vi "create TCPReceiver.vi"(8 "error in (no error)":errorcluster, 10 "Packet Type":refnum<class "TCPPacket.lvclass">, 11 "TCPReceiver in":refnum<class "TCPReceiver.lvclass">) -> (0 "error out":errorcluster, 3 "TCPReceiver out":refnum<class "TCPReceiver.lvclass">)   [LabVIEW 2019, in "TCPReceiver.lvclass"]
uses:
  TCPReceiver.lvclass
  TCPPacket/TCPPacket.lvclass
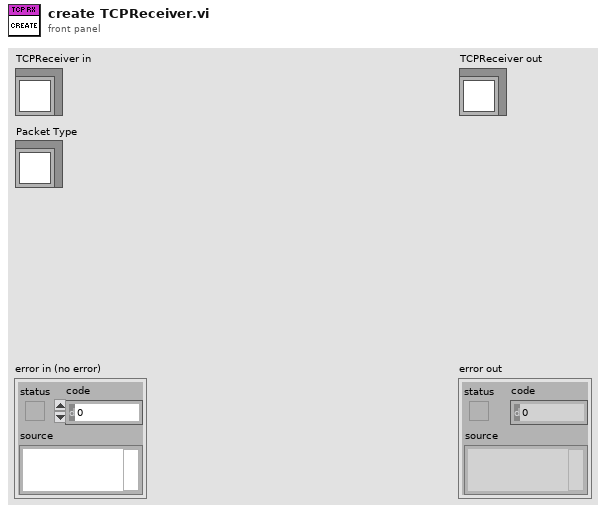
[diagram p1: front panel]
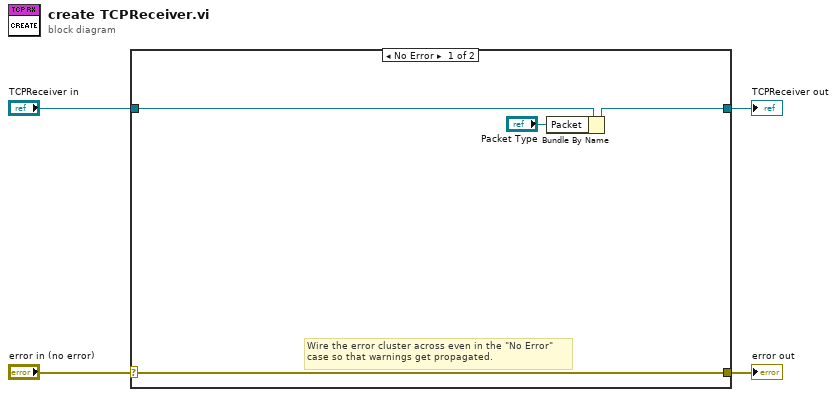
[diagram p0: block diagram]
diagram:
  n1 = case shown="No Error" "error in (no error)" {
    selector: "error in (no error)" -> [w7 w10]
    tunnel: [w7 w10] -> w3
    tunnel: [w6 w9] -> w1
    tunnel: "TCPReceiver in" -> [w8 w9]
    frame No Error {
      # "Wire the error cluster across even in the \"No Error\"\ncase so that warnings get propagated."
      n2 = Bundle By Name(cluster=w8, "Packet"="Packet Type") -> (w6:refnum<class "TCPReceiver.lvclass">)
    }
    frame Error {
    }
  }
  "error out" <- w3
  "TCPReceiver out" <- w1
